vi "Actor Core.vi"(8 "error in":errorcluster, 11 "Table in":refnum<class "Table.lvclass">) -> (0 "error out":errorcluster, 3 "Table out":refnum<class "Actor.lvclass">)   [LabVIEW 2023, in "Table.lvlib" / "Table.lvclass"]
doc: "(<B>Filename</B>: Actor Framework.lvlib:Actor.lvclass:Actor Core.vi)\n\nReceives messages to the actor, reacts to them, and initiates any error handling that may shut the actor down.\n\nDescendant classes may override this VI to append parallel tasks for the actor to complete while it handles messages. Overrides use the Call Parent Method node."
uses:
  Table.lvclass
  C:/Program Files (x86)/National Instruments/LabVIEW 2023/vi.lib/ActorFramework/Actor/Actor.lvclass
  <vilib>/ActorFramework/Actor/Actor.lvclass
  <vilib>/ActorFramework/Actor/Actor.lvclass/Actor.ctl
  <vilib>/ActorFramework/Message Enqueuer/Message Enqueuer.lvclass/Message Enqueuer.ctl
  Table.lvclass/Table.ctl
  Philosopher/Philosopher/Philosopher.lvclass
  Fork State.ctl
  Hungry State.ctl
  <vilib>/ActorFramework/Message Enqueuer/Init from Existing Queue.vi
  <vilib>/ActorFramework/Message Enqueuer/Enqueue.vi
  <vilib>/ActorFramework/Stop Msg/Stop Msg.lvclass
  C:/Program Files (x86)/National Instruments/LabVIEW 2023/vi.lib/ActorFramework/Message/Message.lvclass
  <vilib>/ActorFramework/Message Priority Queue/Priority Enqueue.vi
  <vilib>/ActorFramework/Message Enqueuer/Message Enqueuer.lvclass
panel:
  in  "stop signal":bool
  in  "The End":bool
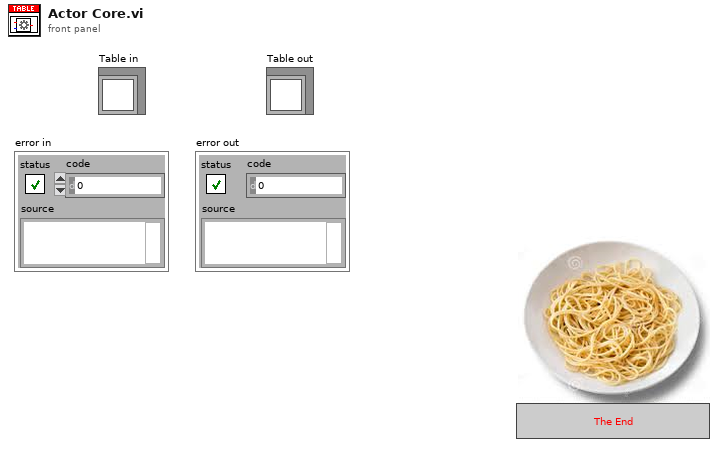
[diagram p1: front panel]
types:
  T1 = typedef "Rendezvous RefNum" = refnum<k1>
  T2 = typedef "Table.lvlib/Table.lvclass/Hungry State.ctl" = enum16{"NO", "YES"}
  T3 = typedef "Table.lvlib/Table.lvclass/Fork State.ctl" = enum16{"FREE", "IN USE"}
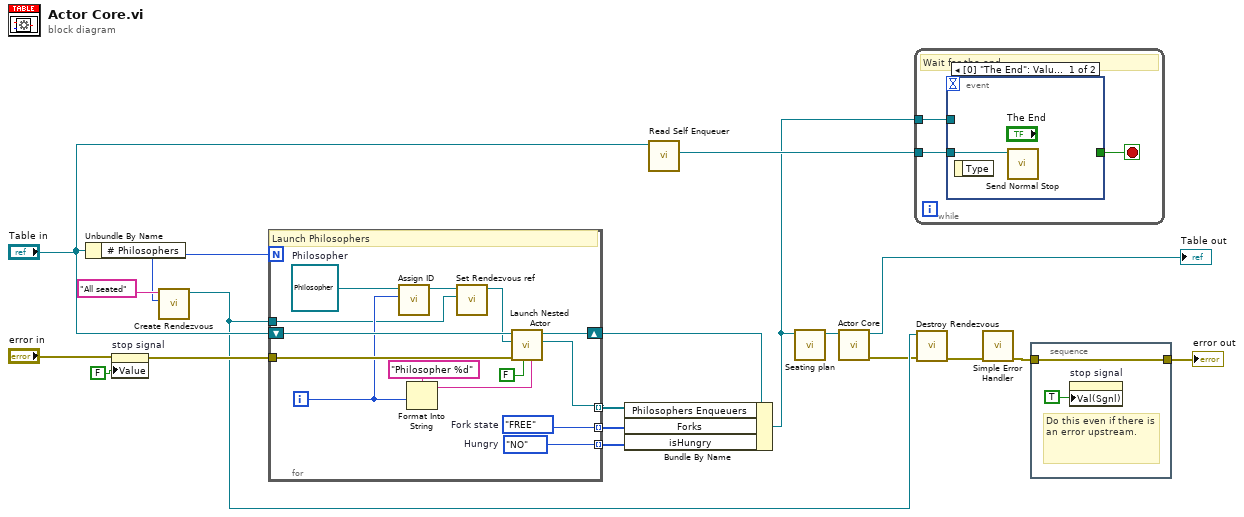
[diagram p0: block diagram]
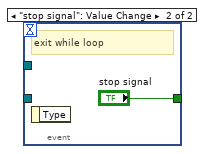
[diagram p2: hidden frame]
diagram:
  n1 = Unbundle By Name("Table in") -> ("# Philosophers"=w4:i32)
  n2 = property on="stop signal" class="Bool (strict)"(error in="error in", "Value"=FALSE ("stop")) -> (error out=w7:errorcluster)  [unwired: 1 in, 1 out]
  n3 = call <vilib>:"Create Rendezvous.vi"("size (2)"=w4, "name (unnamed)"="All seated") -> ("rendezvous"=w2:T1)  [unwired: 3 in, 2 out]
  n4 = for {
    N: w4 -> [_]
    tunnel: w7 -> [w32]
    shift-right: [w30] -> w15
    shift-left: "Table in" -> [w31]
    tunnel: [w29] -> w13 mode=indexing
    tunnel: [w28] -> w12 mode=indexing
    tunnel: [w27] -> w14 mode=indexing
    tunnel: w2 -> [w20]
    i -> [w23]
    w28 = Hungry_State."NO"  # Hungry
    w29 = Fork_State."FREE"  # Fork state
    w24 = refnum<class "Philosopher.lvclass"> refnum  # Philosopher
    # "Launch Philosophers"
    n5 = call-dynamic "Assign ID.vi"("ID"=w23, "Philosopher in"=w24) -> ("Philosopher out"=w22:refnum<class "Philosopher.lvclass">)  [unwired: 8 in, 1 out]
    n6 = Format Into String(format string="Philosopher %d", w23) -> (resulting string=w25:string)  [unwired: 2 in, 1 out]
    n7 = call-dynamic "Set Rendezvous ref.vi"("rendezvous"=w20, "Philosopher in"=w22) -> ("Philosopher out"=w21:refnum<class "Philosopher.lvclass">)  [unwired: 8 in, 1 out]
    n8 = call <vilib>:"Launch Nested Actor.vi"("Debug Alias"=w25, "Open Actor Core front panel? (F)"=FALSE, "error in (no error)"=w32, "Nested Actor"=w21, "Caller Actor in"=w31) -> ("Nested Actor's Enqueuer"=w27:refnum<class "Message Enqueuer.lvclass">, "Caller Actor out"=w30:refnum<class "Table.lvclass">)  [unwired: 4 in, 1 out]
  }
  n9 = Bundle By Name(cluster=w15, "Philosophers Enqueuers"=w14, "Forks"=w13, "isHungry"=w12) -> (w9:refnum<class "Table.lvclass">)
  n10 = call <vilib>:"Read Self Enqueuer.vi"("Actor"="Table in") -> ("Self Enqueuer"=w17:refnum<class "Message Enqueuer.lvclass">)  [unwired: 10 in]
  n11 = call-dynamic "Seating plan.vi"("Table in"=w9) -> ("Table out"=w8:refnum<class "Table.lvclass">)  [unwired: 9 in, 1 out]
  n12 = call-parent "Actor Core.vi"("Actor in"=w8) -> ("error out"=w1:errorcluster, "Actor out"=→"Table out":refnum<class "Actor.lvclass">)  [unwired: 9 in]
  n13 = while {
    tunnel: w17 -> [w36]
    tunnel: w9 -> [w34]
    stop <- w35 stop-if-true
    # "Wait for the end"
    n14 = event shown="[0] \"The End\": Value Change;  Panel Close" {
      selector: _ -> [_ _]
      dyn-events: _ -> [_ _]
      timeout: _ -> [_ _]
      tunnel: w36 -> [w37 _]
      tunnel: [_ "stop signal"] -> w35
      tunnel: w34 -> [_ _]
      event "The End": Value Change; Panel Close {
        n15 = event-data() -> ()  [unwired: 1 in, 1 out]
        n16 = call <vilib>:"Send Normal Stop.vi"("Message Enqueuer"=w37) -> ()  [unwired: 10 in, 1 out]
      }
      event "stop signal": Value Change {
        # "exit while loop"
        n17 = event-data() -> ()  [unwired: 1 in, 1 out]
      }
    }
  }
  n18 = call <vilib>:"Destroy Rendezvous.vi"("error in (no error)"=w1, "rendezvous"=w2) -> ("error out"=w3:errorcluster)  [unwired: 4 in, 1 out]
  n19 = call <vilib>:"Simple Error Handler.vi"("error in (no error)"=w3) -> ("error out"=w16:errorcluster)  [unwired: 4 in, 4 out]
  n20 = stacked-sequence {
    tunnel: [w39] -> w6
    tunnel: w16 -> [w39]
    frame #0 {
      # "Do this even if there is an error upstream."
      n21 = property on="stop signal" class="Bool (strict)"("Val(Sgnl)"=TRUE ("stop")) -> ()  [unwired: 2 in, 2 out]
    }
  }
  "error out" <- w6
